vi "Panel Actor Event Loop.vi"   [LabVIEW 2017]
doc: "Drops a basic template Event Handler Loop that is useful for Panel Actors.\n\n----\nCopyright: MGI 2018\nAuthor: Derek Trepanier"
uses:
  <vilib>/ActorFramework/Stop Msg/Stop Msg.lvclass
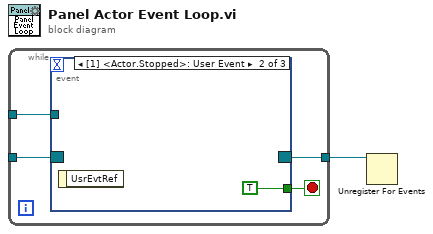
[diagram p0: block diagram]
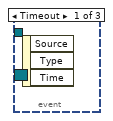
[diagram p2: hidden frame]
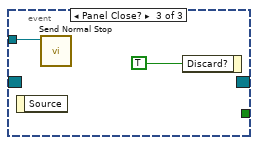
[diagram p3: hidden frame]
diagram:
  n1 = while {
    tunnel: _ -> [w5]
    tunnel: _ -> [w4]
    tunnel: [w2] -> w1
    stop <- w3 stop-if-true
    n2 = event shown="[1] <Actor.Stopped>: User Event" {
      selector: w5 -> [_ _ _]
      dyn-events: [_ _ _] -> w2
      timeout: _ -> [_ _ _]
      tunnel: w4 -> [_ _ w8]
      tunnel: [_ TRUE _] -> w3
      event Timeout {
        n3 = event-data() -> ()  [unwired: 1 in, 3 out]
      }
      event User Event {
        n4 = event-data() -> ()  [unwired: 1 in, 1 out]
      }
      event Panel Close? {
        n5 = event-data() -> ()  [unwired: 1 in, 1 out]
        n6 = call <vilib>:"Send Normal Stop.vi"("Message Enqueuer"=w8) -> ()  [unwired: 10 in, 1 out]
        n7 = event-data("Discard?"=TRUE) -> ()  [unwired: 1 in, 1 out]
      }
    }
  }
  n8 = Unregister For Events(event registration refnum=w1) -> ()  [unwired: 1 in, 1 out]
